vi "Write Box ItemNames.vi"(8 "error in (no error)":errorcluster, 11 "BetterMultiListboxHandle in":refnum<class "BetterMultiListboxHandle.lvclass">) -> (0 "error out":errorcluster, 3 "BetterMultiListboxHandle out":refnum<class "BetterMultiListboxHandle.lvclass">)   [LabVIEW 2020, in "BetterDragAndDrop.lvlib" / "BetterMultiListboxHandle.lvclass"]
uses:
  BetterMultiListboxHandle.lvclass
  C:/DSCE code/Open-source/betterdraganddrop_GIT/Source/Classes/BetterHandle/BetterHandle.lvclass
  BetterHandle/BetterHandle.lvclass/BetterHandle.ctl
  BetterMultiListboxHandle.lvclass/BetterMultiListboxHandle.ctl
  <vilib>/Utility/miscctls.llb/LVRowAndColumnTypeDef.ctl
  BetterTreeItem/BetterItem.lvclass
  BetterHandle/BetterHandle.lvclass
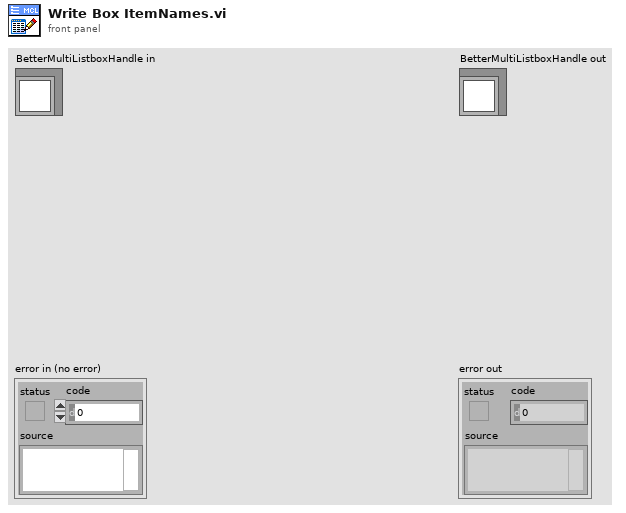
[diagram p1: front panel]
types:
  T1 = typedef "LVRowAndColumnTypeDef.ctl" = cluster{"Row":i32, "Column":i32}
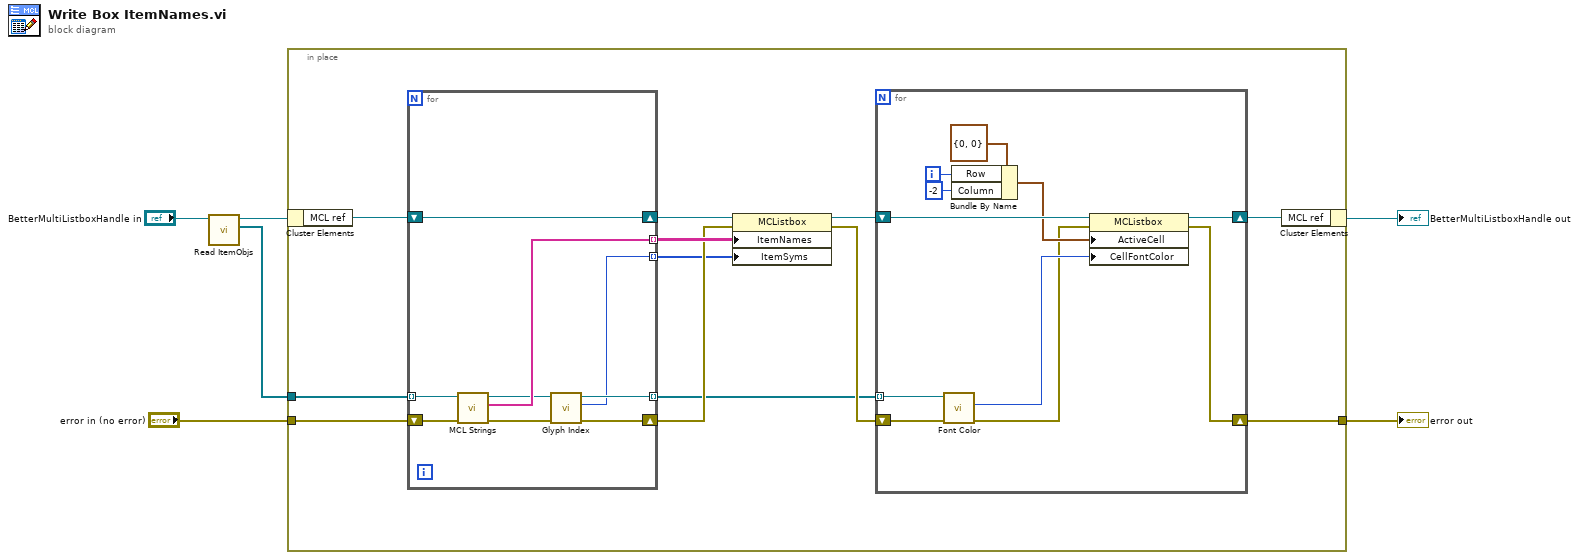
[diagram p0: block diagram]
diagram:
  n1 = call "Read ItemObjs.vi"("BetterHandle in"="BetterMultiListboxHandle in") -> ("ItemObjs"=w4:refnum<class "BetterItem.lvclass">[], "BetterHandle out"=w5:refnum<class "BetterMultiListboxHandle.lvclass">)  [unwired: 9 in]
  n2 = in-place {
    in-place-border: w4 -> [w18]
    in-place-border: "error in (no error)" -> [w16]
    in-place-border: [w9] -> w2
    n3 = in-place-cluster #1(w5) -> ("MCL ref"=w8:refnum<vi>)
    n4 = for {
      tunnel: w18 -> [w38] mode=indexing
      tunnel: [w37] -> w17 mode=indexing
      shift-right: [w32] -> w15
      shift-left: w16 -> [w36]
      tunnel: [w33] -> w12 mode=indexing
      tunnel: [w31] -> w11 mode=indexing
      shift-right: [w30] -> w7
      shift-left: w8 -> [w30]
      n5 = call-dynamic "MCL Strings.vi"("error in (no error)"=w36, "BetterItem in"=w38) -> ("error out"=w34:errorcluster, "Multicolumn Listxox row strings"=w37:string[], "BetterItem out"=w35:refnum<class "BetterItem.lvclass">)  [unwired: 7 in]
      n6 = call-dynamic "Glyph Index.vi"("error in (no error)"=w34, "BetterItem in"=w35) -> ("error out"=w32:errorcluster, "Glyph Index"=w31:i32, "BetterItem out"=w33:refnum<class "BetterItem.lvclass">)  [unwired: 7 in]
    }
    n7 = property class="MCListbox"(reference=w7, error in=w15, "ItemNames"=w17, "ItemSyms"=w11) -> (reference out=w14:refnum<vi>, error out=w13:errorcluster)
    n8 = for {
      shift-right: [w22] -> w10
      shift-left: w14 -> [w26]
      shift-right: [w21] -> w9
      shift-left: w13 -> [w20]
      tunnel: w12 -> [w25] mode=indexing
      i -> [w27]
      n9 = call-dynamic "Font Color.vi"("error in (no error)"=w20, "BetterItem in"=w25) -> ("error out"=w19:errorcluster, "Font Color"=w24:u32)  [unwired: 7 in, 1 out]
      n10 = Bundle By Name(cluster=T1 {"Row"=0, "Column"=0} ("Active Cell:Active Cell"), "Row"=w27, "Column"=-2) -> (w23:T1)
      n11 = property class="MCListbox"(reference=w26, error in=w19, "ActiveCell"=w23, "CellFontColor"=w24) -> (reference out=w22:refnum<vi>, error out=w21:errorcluster)
    }
    n12 = in-place-cluster #1("MCL ref"=w10) -> (→"BetterMultiListboxHandle out":refnum<class "BetterMultiListboxHandle.lvclass">)
  }
  "error out" <- w2
